vi "Concrete Type.vi"(8 "error in (no error)":errorcluster, 11 "Type in":refnum<class "Type.lvclass">) -> (0 "error out":errorcluster, 3 "Concrete Type":refnum<class "Type.lvclass">)   [LabVIEW 2020, in "Conditu2.lvlib" / "Columns.lvlib" / "Type.lvclass"]
uses:
  Type.lvclass
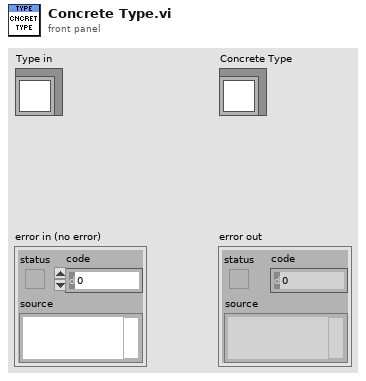
[diagram p1: front panel]
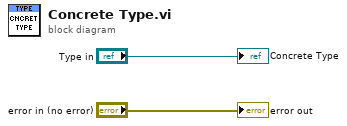
[diagram p0: block diagram]
diagram:
  "error out" <- "error in (no error)"
  "Concrete Type" <- "Type in"
